vi "TCPserverR.vi"(11 "Ref In":T1) -> ()   [LabVIEW 2014]
doc: "Demonstrates how to open a connection to an TCP server, read the data being sent, and display the data on a chart. This VI is designed to stop if the TCP connection is terminated."
panel:
  out "error out":errorcluster
  out "Current Pos":dbl[](array[numeric])
  in  "Position":dbl[](array[numeric])
  in  "Ring":u16(ring) items=["Move2Pos", "Move2Work", "ChangeManipulator", "Move2Home", "Calibration", "CurrentPos", "Interrupt"]
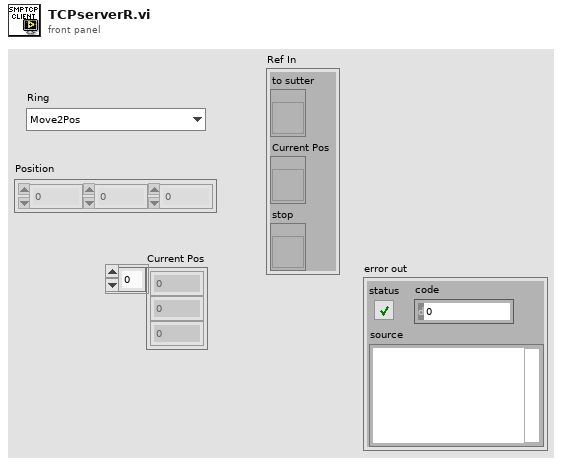
[diagram p1: front panel]
types:
  T1 = cluster{"to sutter":refnum<vi>, "Current Pos":refnum<vi>, "stop":refnum<vi>}
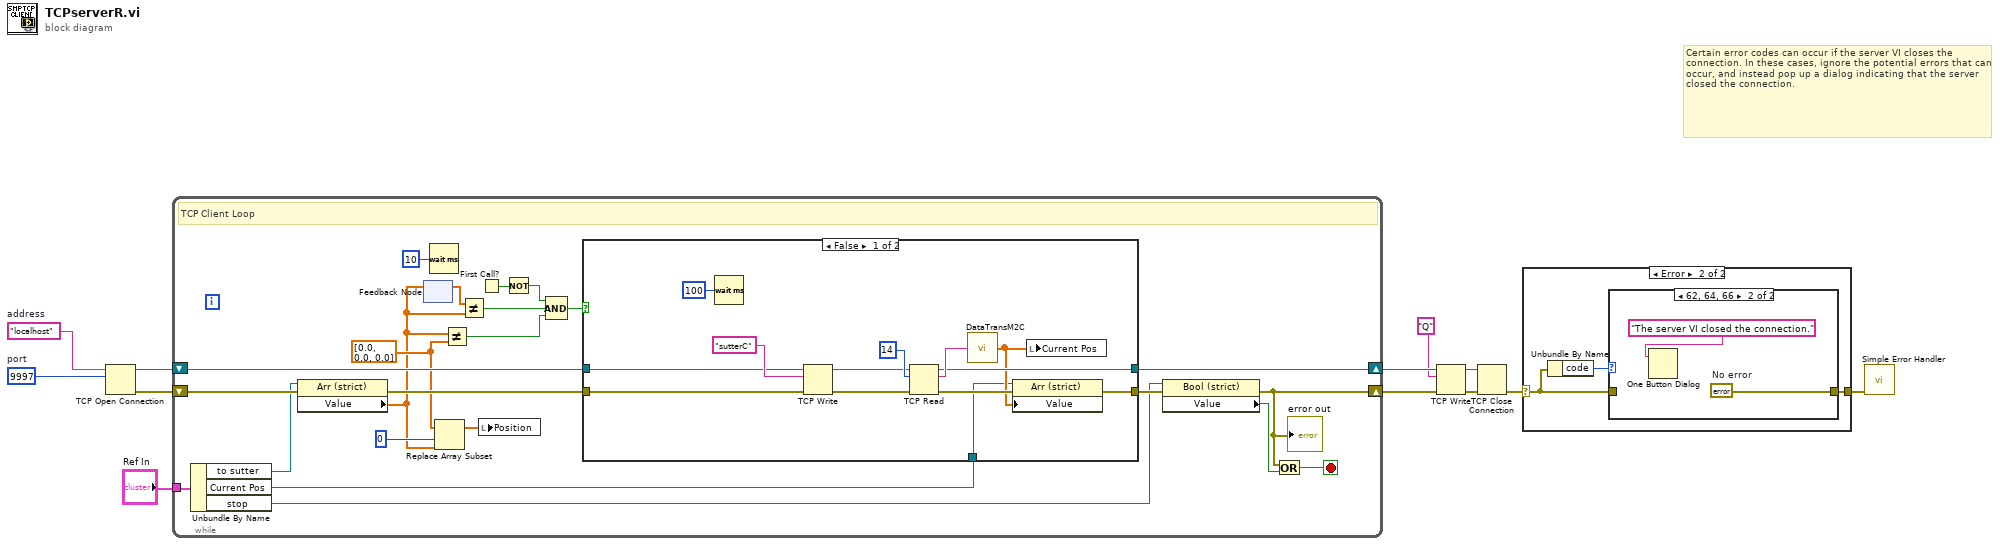
[diagram p0: block diagram]
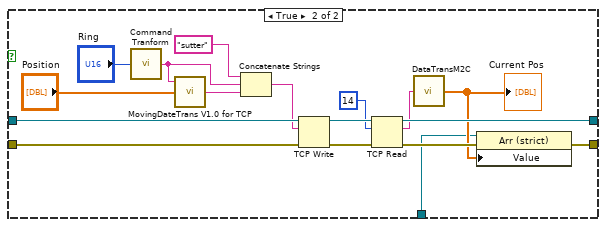
[diagram p4: hidden frame]
diagram:
  w4 = u16 9997  # port
  w5 = "localhost"  # address
  # "Certain error codes can occur if the server VI closes the connection. In these cases, ignore the potential errors that can occur, and instead pop up a dialog indicating that the server closed the connection."
  n1 = TCP Open Connection(address=w5, remote port or service name=w4) -> (connection ID=w2:refnum<k5>, error out=w1:errorcluster)  [unwired: 3 in]
  n2 = while {
    shift-right: [w30] -> w9
    shift-left: w1 -> [w35]
    shift-right: [w32] -> w11
    shift-left: w2 -> [w33]
    tunnel: "Ref In" -> [w27]
    stop <- w34 stop-if-true
    w17 = dbl[] [0.0, 0.0, 0.0] ("x")
    # "TCP Client Loop"
    n3 = Unbundle By Name(w27) -> ("to sutter"=w28:refnum<vi>, "Current Pos"=w22:refnum<vi>, "stop"=w23:refnum<vi>)
    n4 = property class="Arr (strict)"(reference=w28, error in=w35) -> (error out=w19:errorcluster, "Value"=w14:sgl[])  [unwired: 1 out]
    n5 = feedback-in #1(w14) -> ()
    n6 = feedback #1() -> (w15:sgl[])  [unwired: 1 in]
    n7 = Wait (ms)(milliseconds to wait=u32 10) -> ()  [unwired: 1 out]
    n8 = Replace Array Subset(array=w17, new element=w14, index=0) -> (w20:dbl[])
    n9 = Not Equal?(x=w14, y=w17) -> (x != y?=w16:bool)
    n10 = Not Equal?(x=w15, y=w14) -> (x != y?=w13:bool)
    n11 = First Call?() -> (First Call?: T/F=w26:bool)
    n12 = local write "Position"(w20) -> ()
    n13 = Not(x=w26) -> (.not. x?=w25:bool)
    n14 = Compound Arithmetic op=AND(w25, w13, w16) -> (w24:bool)
    n15 = case shown="False" w24 {
      tunnel: w33 -> [w43 w65]
      tunnel: [w41 w64] -> w32
      tunnel: [w39 w51] -> w31
      tunnel: w19 -> [w42 w53]
      tunnel: w22 -> [w37 w49]
      frame False {
        n16 = Wait (ms)(milliseconds to wait=u32 100) -> ()  [unwired: 1 out]
        n17 = TCP Write(connection ID=w43, data in="sutterC", error in (no error)=w42) -> (connection ID out=w46:refnum<k5>, error out=w45:errorcluster)  [unwired: 1 in, 1 out]
        n18 = TCP Read(connection ID=w46, bytes to read=14, error in (no error)=w45) -> (connection ID out=w41:refnum<k5>, data out=w48:string, error out=w40:errorcluster)  [unwired: 2 in]
        n19 = call "DataTransM2C.vi"("MotorData"=w48) -> ("Computer Data"=w38:dbl[])
        n20 = property class="Arr (strict)"(reference=w37, error in=w40, "Value"=w38) -> (error out=w39:errorcluster)  [unwired: 1 out]
        n21 = local write "Current Pos"(w38) -> ()
      }
      frame True {
        n22 = call "Command Tranform.vi"("Command"="Ring") -> ("command str"=w60:string)
        n23 = call "MovingDateTrans V1.0 for TCP.vi"("INPUT"="Position", "String"=w60) -> ("MOVEING COMMAND"=w62:string)  [unwired: 1 in]
        n24 = Concatenate Strings("sutter" ("string"), w60, w62) -> (w55:string)
        n25 = TCP Write(connection ID=w65, data in=w55, error in (no error)=w53) -> (connection ID out=w58:refnum<k5>, error out=w59:errorcluster)  [unwired: 1 in, 1 out]
        n26 = TCP Read(connection ID=w58, bytes to read=14, error in (no error)=w59) -> (connection ID out=w64:refnum<k5>, data out=w56:string, error out=w52:errorcluster)  [unwired: 2 in]
        n27 = call "DataTransM2C.vi"("MotorData"=w56) -> ("Computer Data"=w50:dbl[])
        "Current Pos" <- w50
        n28 = property class="Arr (strict)"(reference=w49, error in=w52, "Value"=w50) -> (error out=w51:errorcluster)  [unwired: 1 out]
      }
    }
    n29 = property class="Bool (strict)"(reference=w23, error in=w31) -> (error out=w30:errorcluster, "Value"=w29:bool)  [unwired: 1 out]
    "error out" <- w30
    n30 = Or(x=w30, y=w29) -> (x .or. y?=w34:bool)
  }
  n31 = TCP Write(connection ID=w11, data in="Q", error in (no error)=w9) -> (connection ID out=w12:refnum<k5>, error out=w10:errorcluster)  [unwired: 2 out]
  n32 = TCP Close Connection(connection ID=w12, error in (no error)=w10) -> (error out=w7:errorcluster)  [unwired: 1 in, 1 out]
  n33 = case shown="Error" w7 {
    selector: w7 -> [w66 w68]
    tunnel: [w66 w67] -> w6
    frame No Error {
    }
    frame Error {
      n34 = Unbundle By Name(w68) -> ("code"=w69:i32)
      n35 = case shown="62, 64, 66" w69 {
        tunnel: w68 -> [w70 _]
        tunnel: [w70 w72] -> w67
        frame Default {
        }
        frame 62, 64, 66 {
          w72 = errorcluster {"status"=FALSE, "code"=0, "source"=""}  # No error
          n36 = One Button Dialog(message="The server VI closed the connection.") -> ()  [unwired: 1 in, 1 out]
        }
      }
    }
  }
  n37 = call <vilib>:"Simple Error Handler.vi"("error in (no error)"=w6) -> ()  [unwired: 4 in, 5 out]
